vi "Stop Work.vi"(8 "error in (no error)":errorcluster, 9 "Reply":bool=TRUE, 10 "Reply to":refnum<class "Stop Response Msg.lvclass">, 11 "Measure Object in":refnum<class "Process Object.lvclass">) -> (0 "error out":errorcluster, 3 "Measure Object out":refnum<class "Process Object.lvclass">)   [LabVIEW 2018, in "Process Object.lvclass"]
uses:
  Process Object.lvclass
  C:/Program Files/National Instruments/LabVIEW 2018/vi.lib/ActorFramework/Actor/Actor.lvclass
  Controllers/Process Controller Messages/Stop Response Msg/Stop Response Msg.lvclass
  Process Object.lvclass/Process Object.ctl
  <vilib>/ActorFramework/Actor/Actor.lvclass/Actor.ctl
  <vilib>/ActorFramework/Message Enqueuer/Message Enqueuer.lvclass/Message Enqueuer.ctl
  Template Module Messages/Unubscribe Request Msg/Unubscribe Request Msg.lvclass/Unubscribe Request Msg.ctl
  Read Broadcaster name.vi
  <vilib>/ActorFramework/Message Enqueuer/Init from Existing Queue.vi
  <vilib>/ActorFramework/Message Enqueuer/Enqueue.vi
  Template Module Messages/Unubscribe Request Msg/Unubscribe Request Msg.lvclass
  C:/Program Files/National Instruments/LabVIEW 2018/vi.lib/ActorFramework/Message/Message.lvclass
  <vilib>/ActorFramework/Message Priority Queue/Priority Enqueue.vi
  Worker/Worker.lvclass
  <vilib>/ActorFramework/Message Enqueuer/Message Enqueuer.lvclass
  <vilib>/ActorFramework/Actor/Actor.lvclass
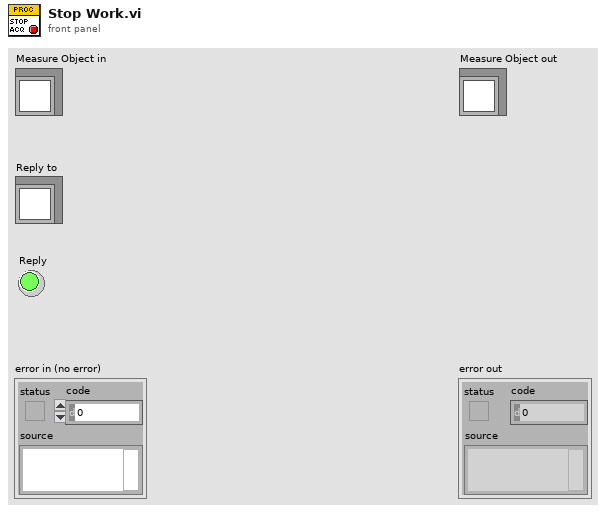
[diagram p1: front panel]
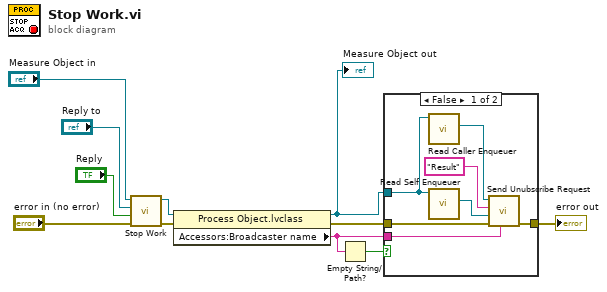
[diagram p0: block diagram]
diagram:
  n1 = call-parent "Stop Work.vi"("error in (no error)"="error in (no error)", "Reply"="Reply", "Reply to"="Reply to", "Measure Object in"="Measure Object in") -> ("error out"=w3:errorcluster, "Measure Object out"=w5:refnum<class "Process Object.lvclass">)  [unwired: 6 in]
  n2 = property class="Process Object.lvclass"(reference=w5, error in=w3) -> (reference out=w4:refnum<class "Process Object.lvclass">, error out=w6:errorcluster, "Accessors:Broadcaster name"=w1:string)
  "Measure Object out" <- w4
  n3 = Empty String/Path?(string/path=w1) -> (empty?=w7:bool)
  n4 = case shown="False" w7 {
    tunnel: w6 -> [w18 w19]
    tunnel: [w14 w19] -> w2
    tunnel: w4 -> [w13 _]
    tunnel: w1 -> [w12 _]
    frame False {
      n5 = call <vilib>:"Read Caller Enqueuer.vi"("Actor"=w13) -> ("Caller Enqueuer"=w16:refnum<class "Message Enqueuer.lvclass">)  [unwired: 10 in]
      n6 = call <vilib>:"Read Self Enqueuer.vi"("Actor"=w13) -> ("Self Enqueuer"=w17:refnum<class "Message Enqueuer.lvclass">)  [unwired: 10 in]
      n7 = call "Send Unubscribe Request.vi"("Broadcaster"=w12, "error in (no error)"=w18, "Subscriber Enqueuer"=w17, "Topic"="Result", "Message Enqueuer"=w16) -> ("error out"=w14:errorcluster)  [unwired: 5 in, 1 out]
    }
    frame True {
    }
  }
  "error out" <- w2
